vi "Read Menu Action.vi"(8 "error in (no error)":errorcluster, 10 "ItemTag":string, 11 "MLA in":refnum<class "MLA.lvclass">) -> (0 "error out":errorcluster, 3 "MLA out":refnum<class "MLA.lvclass">)   [LabVIEW 2017]
uses:
  MLA/MLA.lvclass
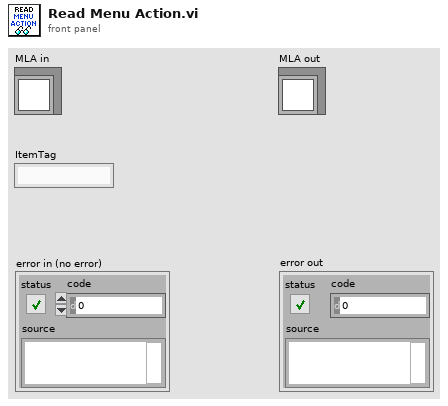
[diagram p1: front panel]
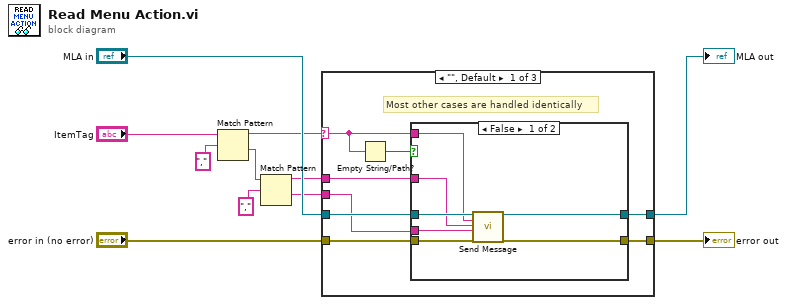
[diagram p0: block diagram]
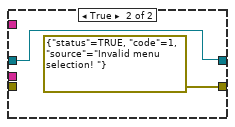
[diagram p2: hidden frame]
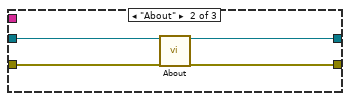
[diagram p3: hidden frame]
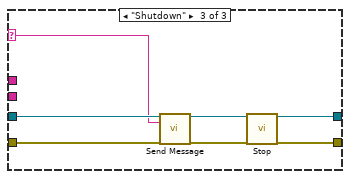
[diagram p4: hidden frame]
diagram:
  n1 = Match Pattern(string="ItemTag", regular expression=",") -> (before substring=w5:string, after substring=w6:string)  [unwired: 1 in, 2 out]
  n2 = Match Pattern(string=w6, regular expression=",") -> (before substring=w4:string, after substring=w3:string)  [unwired: 1 in, 2 out]
  n3 = case shown="\"\", Default" w5 {
    selector: w5 -> [w14 _ w33]
    tunnel: "error in (no error)" -> [w19 w32 w39]
    tunnel: [w18 w31 w36] -> w2
    tunnel: "MLA in" -> [w17 w29 w37]
    tunnel: [w16 w30 w34] -> w1
    tunnel: w4 -> [w15 _ _]
    tunnel: w3 -> [w12 _ _]
    frame "", Default {
      # "Most other cases are handled identically"
      n4 = Empty String/Path?(string/path=w14) -> (empty?=w13:bool)
      n5 = case shown="False" w13 {
        tunnel: w19 -> [w26 _]
        tunnel: [w25 errorcluster {"status"=TRUE, "code"=1, "source"="Invalid menu selection! "} ("error constant")] -> w18
        tunnel: w17 -> [w24 w27]
        tunnel: [w23 w27] -> w16
        tunnel: w14 -> [w22 _]
        tunnel: w15 -> [w21 _]
        tunnel: w12 -> [w20 _]
        frame False {
          n6 = call-dynamic "Send Message.vi"("MLA"=w24, "Message"=w22, "Param 1"=w21, "Param 2"=w20, "error in (no error)"=w26) -> ("MLA"=w23:refnum<class "MLA.lvclass">, "error out"=w25:errorcluster)  [unwired: 13 in]
        }
        frame True {
        }
      }
    }
    frame "About" {
      n7 = call "About.vi"("MLA"=w29, "error in (no error)"=w32) -> ("MLA"=w30:refnum<class "MLA.lvclass">, "error out"=w31:errorcluster)  [unwired: 15 in, 1 out]
    }
    frame "Shutdown" {
      n8 = call-dynamic "Send Message.vi"("MLA"=w37, "Message"=w33, "error in (no error)"=w39) -> ("MLA"=w35:refnum<class "MLA.lvclass">, "error out"=w38:errorcluster)  [unwired: 15 in]
      n9 = call-dynamic "Stop.vi"("reference in"=w35, "error in (no error)"=w38) -> ("reference out"=w34:refnum<class "MLA.lvclass">, "error out"=w36:errorcluster)  [unwired: 16 in]
    }
  }
  "MLA out" <- w1
  "error out" <- w2
